vi "DAQmx Query.vi"() -> (0 "error out":errorcluster, 1 "Serial Number":string[](array[string]), 2 "Error?":bool[](array[boolean]), 3 "Array":T1(array[cluster]), 4 "Product Category":string[](array[string]), 5 "Device Name":string[](array[string]), 6 "Product Type":string[](array[string]), 7 "Simulated?":bool[](array[boolean]), 8 "DO.Lines":tag[](array[tag]))   [LabVIEW 2014, in "SetUp VIs.lvlib"]
uses:
  SetUp VIs.lvlib
  <resource>/objmgr/daqmx.rc
panel:
  out "index of element":i32
  out "Match":string
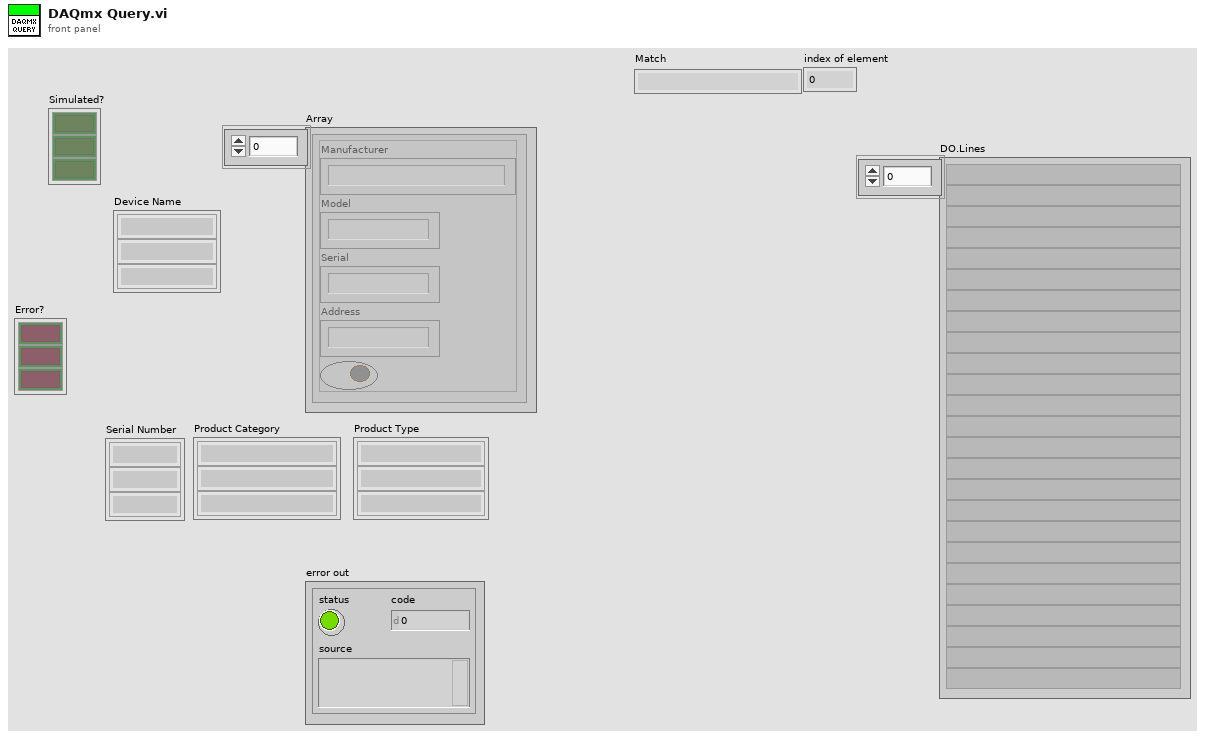
[diagram p1: front panel]
types:
  T1 = cluster{"Manufacturer":string, "Model":string, "Serial":string, "Address":string, "Boolean":bool}[]
  T2 = cluster{"Manufacturer":string, "Model":string, "Serial":string, "Address":string, bool}
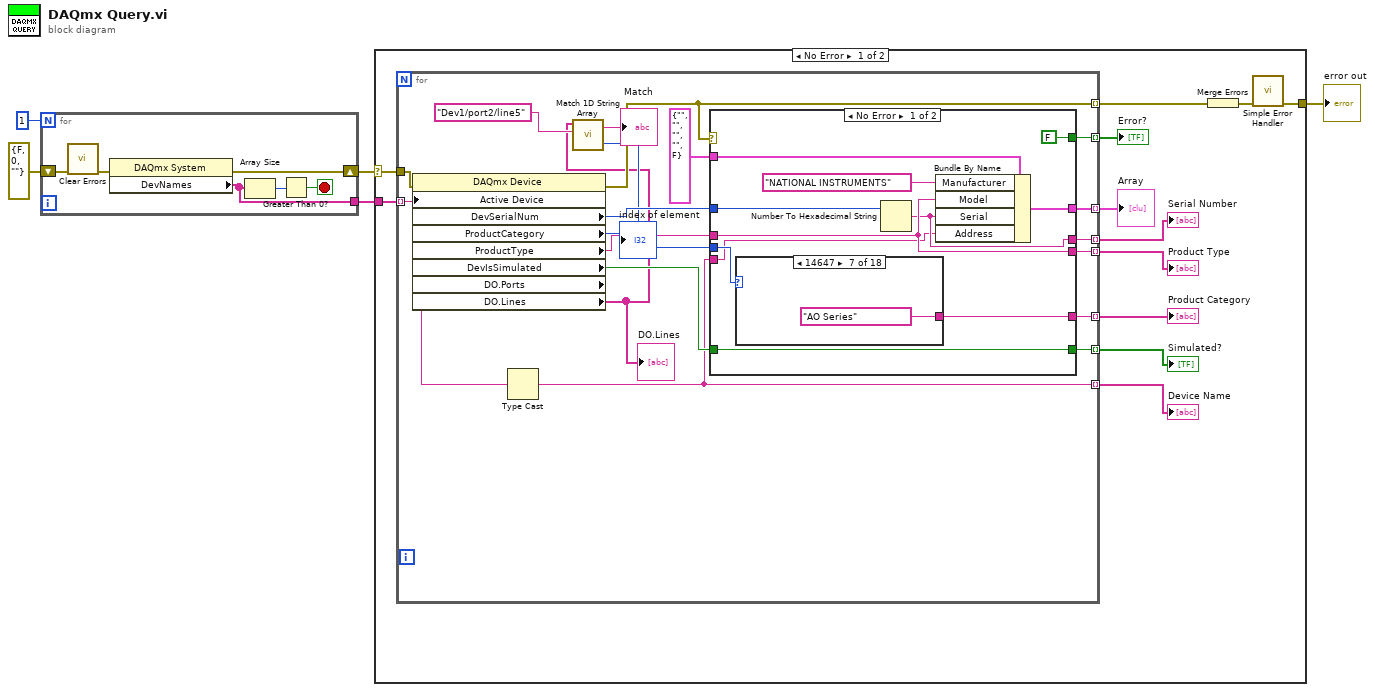
[diagram p0: block diagram]
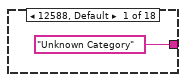
[diagram p2: hidden frame]
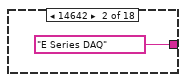
[diagram p3: hidden frame]
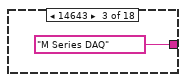
[diagram p4: hidden frame]
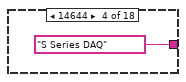
[diagram p5: hidden frame]
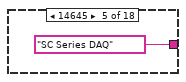
[diagram p6: hidden frame]
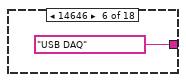
[diagram p7: hidden frame]
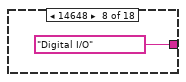
[diagram p8: hidden frame]
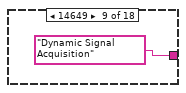
[diagram p9: hidden frame]
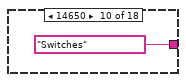
[diagram p10: hidden frame]
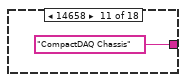
[diagram p11: hidden frame]
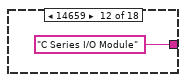
[diagram p12: hidden frame]
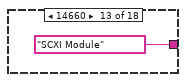
[diagram p13: hidden frame]
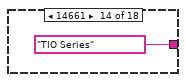
[diagram p14: hidden frame]
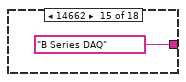
[diagram p15: hidden frame]
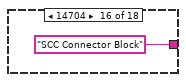
[diagram p16: hidden frame]
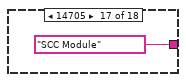
[diagram p17: hidden frame]
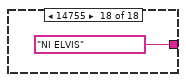
[diagram p18: hidden frame]
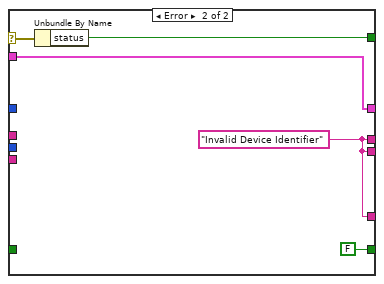
[diagram p19: hidden frame]
diagram:
  n1 = for {
    N: 1 -> [_]
    tunnel: [w8] -> w4
    shift-right: [w11] -> w1
    shift-left: errorcluster {"status"=FALSE, "code"=0, "source"=""} ("error out") -> [w10]
    stop <- w6 stop-if-true
    n2 = call <vilib>:"Clear Errors.vi"("error in (no error)"=w10) -> ("error out"=w9:errorcluster)  [unwired: 5 in, 1 out]
    n3 = property class="DAQmx System"(error in=w9) -> (error out=w11:errorcluster, "DevNames"=w8:tag[])  [unwired: 1 in, 1 out]
    n4 = Array Size(array=w8) -> (size(s)=w7:i32)
    n5 = Greater Than 0?(x=w7) -> (x > 0?=w6:bool)
  }
  n6 = case shown="No Error" w1 {
    selector: w1 -> [w12 w77]
    tunnel: [w23 w77] -> w5
    tunnel: w4 -> [w21 _]
    frame No Error {
      n7 = for {
        tunnel: w21 -> [w39] mode=indexing
        tunnel: [w33] -> w19 mode=indexing
        tunnel: [w40] -> w20 mode=indexing
        tunnel: [w35] -> w18 mode=indexing
        tunnel: [w28] -> w17 mode=indexing
        tunnel: [w37] -> w16 mode=indexing
        tunnel: w12 -> [w42]
        tunnel: [w32] -> w15 mode=indexing
        tunnel: [w31] -> w14 mode=indexing
        tunnel: [w30] -> w22 mode=indexing
        n8 = property class="DAQmx Device" props=["Active Device", "DevSerialNum", "ProductCategory", "ProductType", "DevIsSimulated", "DO.Ports", "DO.Lines"](error in=w42, "Active Device"=w39) -> (error out=w31:errorcluster, "DevSerialNum"=w38:u32, "ProductCategory"=w41:i32, "ProductType"=w34:string, "DevIsSimulated"=w36:bool, "DO.Lines"=w24:tag[])  [unwired: 1 in, 2 out]
        "DO.Lines" <- w24
        n9 = Type Cast(x=w39) -> (*(type *) &x=w28:string)  [unwired: 1 in]
        n10 = call <vilib>:"Match 1D String Array.vi"("Pattern"="Dev1/port2/line5" ("concatenated string"), "Strings"=w24) -> ("index of element"=→"index of element":i32, "Match"=→"Match":string)  [unwired: 2 in]
        n11 = case shown="No Error" w31 {
          selector: w31 -> [_ w73]
          tunnel: w41 -> [w53 _]
          tunnel: [w52 w75] -> w40
          tunnel: w38 -> [w51 _]
          tunnel: [w46 w75] -> w37
          tunnel: w36 -> [w50 _]
          tunnel: [w50 FALSE ("DevIsSimulated")] -> w35
          tunnel: w34 -> [w47 _]
          tunnel: [w47 w75] -> w33
          tunnel: [FALSE ("status") w74] -> w32
          tunnel: [w45 w72] -> w30
          tunnel: T2 {"Manufacturer"="", "Model"="", "Serial"="", "Address"="", FALSE} ("Instrument") -> [w44 w72]
          tunnel: w28 -> [w43 _]
          frame No Error {
            n12 = case shown="14647" w53 {
              tunnel: ["Unknown Category" "E Series DAQ" "M Series DAQ" "S Series DAQ" "SC Series DAQ" "USB DAQ" "AO Series" "Digital I/O" "Dynamic Signal Acquisition" "Switches" "CompactDAQ Chassis" "C Series I/O Module" "SCXI Module" "TIO Series" "B Series DAQ" "SCC Connector Block" "SCC Module" "NI ELVIS"] -> w52
              frame 12588, Default {
              }
              frame 14642 {
              }
              frame 14643 {
              }
              frame 14644 {
              }
              frame 14645 {
              }
              frame 14646 {
              }
              frame 14647 {
              }
              frame 14648 {
              }
              frame 14649 {
              }
              frame 14650 {
              }
              frame 14658 {
              }
              frame 14659 {
              }
              frame 14660 {
              }
              frame 14661 {
              }
              frame 14662 {
              }
              frame 14704 {
              }
              frame 14705 {
              }
              frame 14755 {
              }
            }
            n13 = Number To Hexadecimal String(2:w51) -> (0:w46:string)  [unwired: 1 in]
            n14 = Bundle By Name(cluster=w44, "Manufacturer"="NATIONAL INSTRUMENTS", "Model"=w47, "Serial"=w46, "Address"=w43) -> (w45:T2)
          }
          frame Error {
            w75 = "Invalid Device Identifier"
            n15 = Unbundle By Name(w73) -> ("status"=w74:bool)
          }
        }
      }
      "Product Category" <- w20
      "Product Type" <- w19
      "Simulated?" <- w18
      "Device Name" <- w17
      "Serial Number" <- w16
      "Error?" <- w15
      "Array" <- w22
      n16 = Merge Errors(w14) -> (w13:errorcluster)
      n17 = call <vilib>:"Simple Error Handler.vi"("error in (no error)"=w13) -> ("error out"=w23:errorcluster)  [unwired: 4 in, 4 out]
    }
    frame Error {
    }
  }
  "error out" <- w5
